vi "Send Message.vi"(8 "error in (no error)":errorcluster, 11 "Message Type in":refnum<class "Message Type.lvclass">) -> (0 "error out":errorcluster, 3 "Message Type out":refnum<class "Message Type.lvclass">)   [LabVIEW 2023, in "Message Type.lvclass"]
uses:
  Message Type.lvclass
  Message Type.lvclass/Message Type.ctl
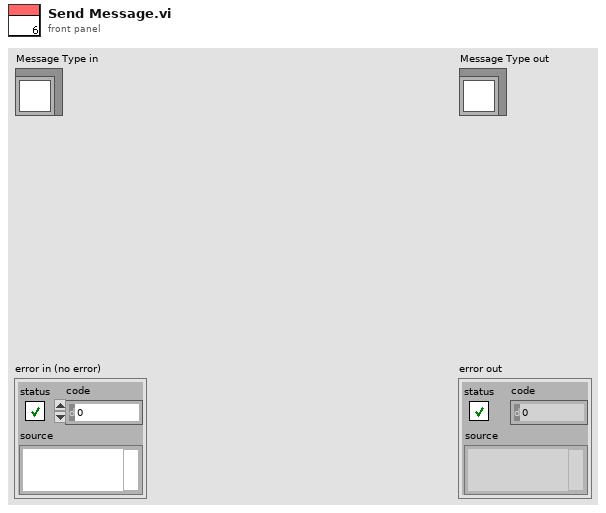
[diagram p1: front panel]
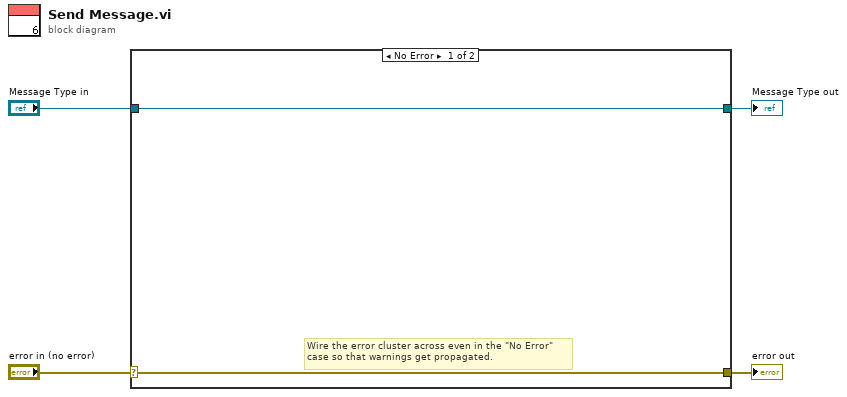
[diagram p0: block diagram]
diagram:
  n1 = case shown="No Error" "error in (no error)" {
    selector: "error in (no error)" -> [w5 w8]
    tunnel: [w5 w8] -> w3
    tunnel: [w6 w7] -> w1
    tunnel: "Message Type in" -> [w6 w7]
    frame No Error {
      # "Wire the error cluster across even in the \"No Error\"\ncase so that warnings get propagated."
    }
    frame Error {
    }
  }
  "error out" <- w3
  "Message Type out" <- w1
